vi "LocalGoal_Msg.vi"(8 "error in (no error)":errorcluster caption="错误输入（无错误）", 10 "值(信号)":T1, 11 "States.lvlib:Guide.lvclass":refnum<class "Guide.lvclass">) -> (0 "error out":errorcluster caption="错误输出", 3 "Process State out":refnum<class "State Actor.lvclass">)   [LabVIEW 2014, in "States.lvlib" / "Guide.lvclass"]
uses:
  Guide.lvclass
  <vilib>/NI/Actors/State Actor/State Actor/State Actor.lvclass
  ctl/Point.ctl
  <vilib>/ActorFramework/Message Enqueuer/Message Enqueuer.lvclass/Message Enqueuer.ctl
  <vilib>/ActorFramework/Message Enqueuer/Enqueue.vi
  <vilib>/ActorFramework/Message Priority Queue/Priority Enqueue.vi
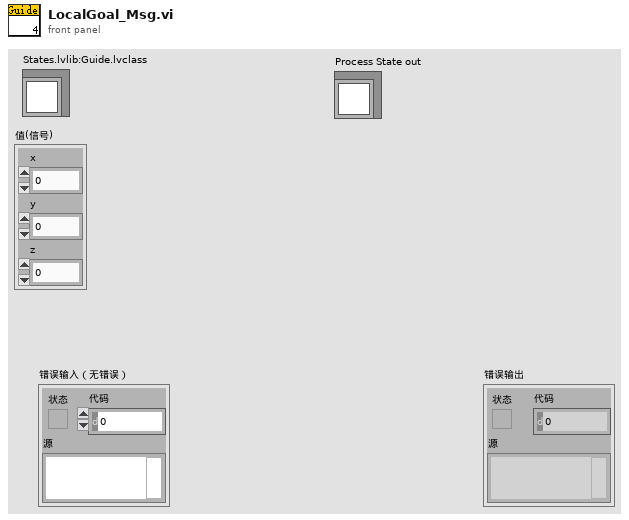
[diagram p1: front panel]
types:
  T1 = typedef "Point.ctl" = cluster{"x":dbl, "y":dbl, "z":dbl}
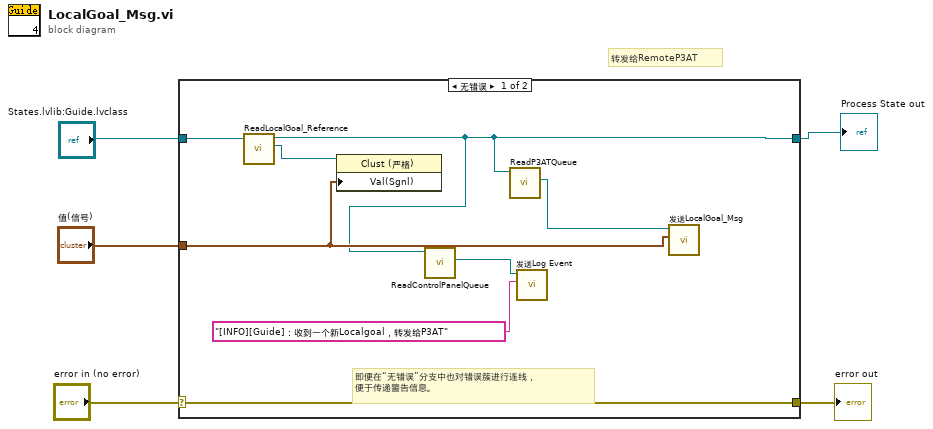
[diagram p0: block diagram]
diagram:
  # "转发给RemoteP3AT"
  n1 = case shown="无错误" "error in (no error)" {
    selector: "error in (no error)" -> [w13 w15]
    tunnel: [w13 w15] -> w4
    tunnel: [w6 w14] -> w3
    tunnel: "States.lvlib:Guide.lvclass" -> [w12 w14]
    tunnel: "值(信号)" -> [w9 _]
    frame No Error {
      # "即便在“无错误”分支中也对错误簇进行连线，\n便于传递警告信息。"
      n2 = call-dynamic "ReadLocalGoal_Reference.vi"("CoordinatorState输入"=w12) -> ("LocalGoal_Reference"=w11:refnum<vi>, "CoordinatorState输出"=w6:refnum<class "Guide.lvclass">)  [unwired: 8 in, 1 out]
      n3 = property class="Clust (严格)"(reference=w11, "Val(Sgnl)"=w9) -> ()  [unwired: 1 in, 2 out]
      n4 = call-dynamic "ReadControlPanelQueue.vi"("CoordinatorState输入"=w6) -> ("操作者框架:消息待入队列"=w7:refnum<class "Message Enqueuer.lvclass">)  [unwired: 8 in, 2 out]
      n5 = call-dynamic "ReadP3ATQueue.vi"("CoordinatorState输入"=w6) -> ("操作者框架:消息待入队列"=w10:refnum<class "Message Enqueuer.lvclass">)  [unwired: 8 in, 2 out]
      n6 = call "发送Log Event.vi"("Event Text"="[INFO][Guide]：收到一个新Localgoal，转发给P3AT", "消息待入队列"=w7) -> ()  [unwired: 8 in, 2 out]
      n7 = call "发送LocalGoal_Msg.vi"("值(信号)"=w9, "消息待入队列"=w10) -> ()  [unwired: 8 in, 2 out]
    }
    frame Error {
    }
  }
  "error out" <- w4
  "Process State out" <- w3
